vi "Modify_Image_Thresholding_Settings-1.vi"(4 "[IN] Filtering Settings":T1, 5 "[IN] Index for thresholding 2":u8, 6 "[IN] Sigma #2":dbl min=0.1, 7 "[IN] Index for thresholding":u8, 8 "[IN] Sigma":dbl min=0.1) -> (2 "[OUT] Filtering Settings":T1)   [LabVIEW 2013]
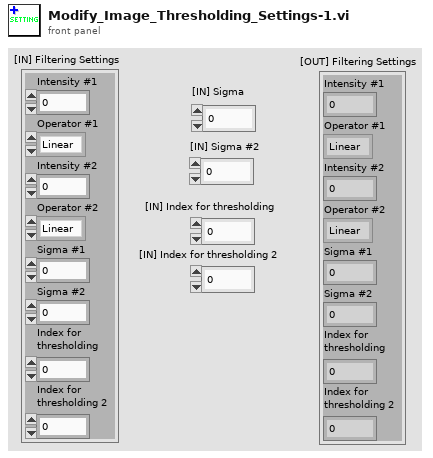
[diagram p1: front panel]
types:
  T1 = cluster{"Intensity #1":sgl, "Operator #1":enum32{"Linear", "Log", "Exp", "Square", "Square root", "Power X", "Power 1/X"}, "Intensity #2":sgl, "Operator #2":enum32{"Linear", "Log", "Exp", "Square", "Square root", "Power X", "Power 1/X"}, "Sigma #1":dbl, "Sigma #2":dbl, "Index for \nthresholding":u8, "Index for \nthresholding 2":u8}
  T2 = enum32{"Linear", "Log", "Exp", "Square", "Square root", "Power X", "Power 1/X"}
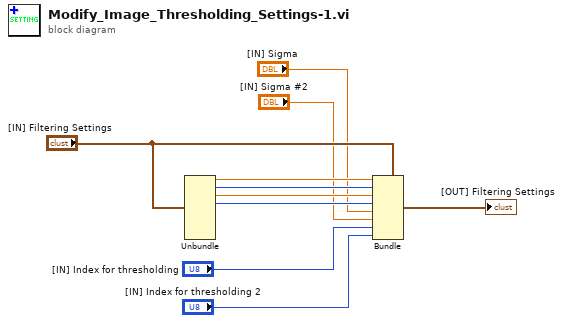
[diagram p0: block diagram]
diagram:
  n1 = Unbundle("[IN] Filtering Settings") -> ("Intensity #1"=w9:sgl, "Operator #1"=w8:T2, "Intensity #2"=w7:sgl, "Operator #2"=w6:T2)  [unwired: 4 out]
  n2 = Bundle(cluster="[IN] Filtering Settings", "Intensity #1"=w9, "Operator #1"=w8, "Intensity #2"=w7, "Operator #2"=w6, "Sigma #1"="[IN] Sigma", "Sigma #2"="[IN] Sigma #2", "Index for \nthresholding"="[IN] Index for thresholding", "Index for \nthresholding 2"="[IN] Index for thresholding 2") -> (→"[OUT] Filtering Settings":T1)
